vi "dotNET Decompress String.vi"(8 "error in (no error)":errorcluster, 11 "GZIP Compressed String":string) -> (0 "error out":errorcluster, 3 "Uncompressed String":string)   [LabVIEW 2010]
doc: "Decompresses the input string using the gzip standard. \n\nOutput is a standard string.\n\nUses: reduce load on transport of data between LabVIEW nodes, saved to save storage space on disk or in a database, obfuscate the contents of a message or file (cheesey encryption).\n\nThis VI makes use of the .NET 2.0 framework.\n\nREV 1.0.0 10/02/2009 P.Brooks\n Originated."
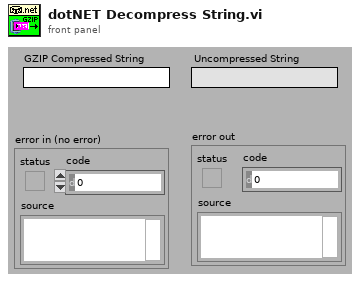
[diagram p1: front panel]
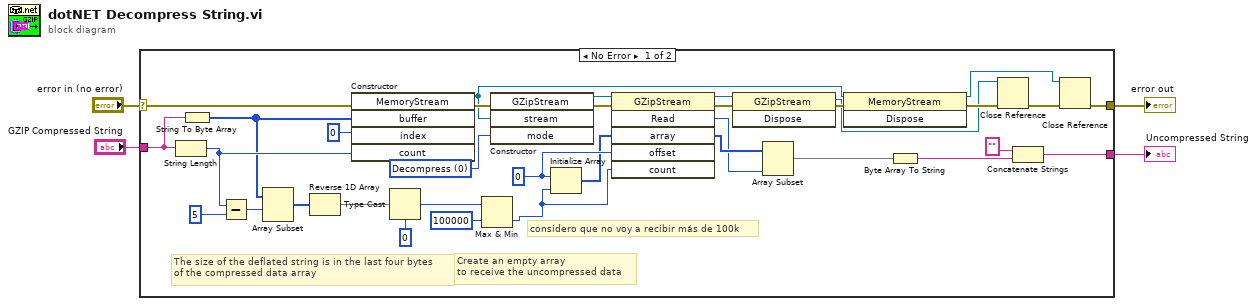
[diagram p0: block diagram]
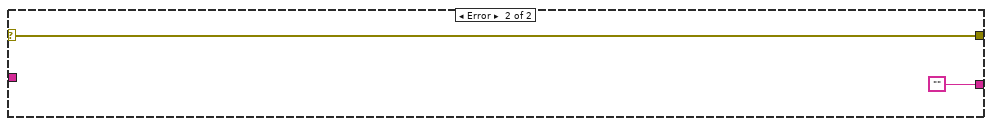
[diagram p2: hidden frame]
diagram:
  n1 = case shown="No Error" "error in (no error)" {
    selector: "error in (no error)" -> [w10 w40]
    tunnel: "GZIP Compressed String" -> [w8 _]
    tunnel: [w31 ""] -> w3
    tunnel: [w14 w40] -> w2
    frame No Error {
      w20 = u8 0 ("offset")
      w23 = 0 items=["Decompress", "Compress"] ("mode")
      # "considero que no voy a recibir más de 100k"
      # "Create an empty array \nto receive the uncompressed data"
      # "The size of the deflated string is in the last four bytes \nof the compressed data array"
      n2 = String Length(string=w8) -> (length=w32:i32)
      n3 = String To Byte Array(string=w8) -> (unsigned byte array=w9:u8[])
      n4 = Subtract(x=w32, y=5) -> (x-y=w34:i32)
      n5 = Array Subset(array=w9, index=w34) -> (w35:u8[])  [unwired: 1 in]
      n6 = Reverse 1D Array(array=w35) -> (reversed array=w36:u8[])
      n7 = constructor class="MemoryStream"(error in=w10, "buffer"=w9, "index"=0, "count"=w32) -> (reference out=w22:refnum<k24>, error out=w38:errorcluster)  [unwired: 2 in, 4 out]
      n8 = Type Cast(type=u32 0, x=w36) -> (*(type *) &x=w7:u32)
      n9 = Max & Min(x=w7, y=u32 100000) -> (min(x,y)=w5:u32)  [unwired: 1 out]
      n10 = constructor class="GZipStream"(error in=w38, "stream"=w22, "mode"=w23) -> (reference out=w25:refnum<k24>, error out=w26:errorcluster)  [unwired: 2 in, 3 out]
      n11 = Initialize Array(w20, w5) -> (w19:u8[])
      n12 = invoke class="GZipStream" method="Read"(reference=w25, error in=w26, "array"=w19, "offset"=w20, "count"=w5) -> (reference out=w24:refnum<k24>, error out=w27:errorcluster, "Read"=w16:i32, "array"=w21:u8[])  [unwired: 1 in, 2 out]
      n13 = invoke class="GZipStream" method="Dispose"(reference=w24, error in=w27) -> (reference out=w11:refnum<k24>, error out=w28:errorcluster)  [unwired: 1 in, 1 out]
      n14 = Array Subset(array=w21, length=w16) -> (w17:u8[])  [unwired: 1 in]
      n15 = invoke class="MemoryStream" method="Dispose"(reference=w22, error in=w28) -> (reference out=w15:refnum<k24>, error out=w13:errorcluster)  [unwired: 1 in, 1 out]
      n16 = Byte Array To String(unsigned byte array=w17) -> (string=w18:string)
      n17 = Close Reference(reference=w11, error in (no error)=w13) -> (error out=w12:errorcluster)
      n18 = Concatenate Strings("", w18) -> (w31:string)
      n19 = Close Reference(reference=w15, error in (no error)=w12) -> (error out=w14:errorcluster)
    }
    frame Error {
    }
  }
  "Uncompressed String" <- w3
  "error out" <- w2
